vi "RollCalc.vi"(10 "Previous Roll Value":dbl, 11 "Roll Input":dbl) -> (2 "New Roll Value":dbl, 3 "Adjustment to be Made":dbl)   [LabVIEW 2015, in "lv-attitudecontrol.lvlib"]
uses:
  lv-attitudecontrol.lvlib
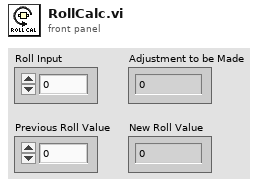
[diagram p1: front panel]
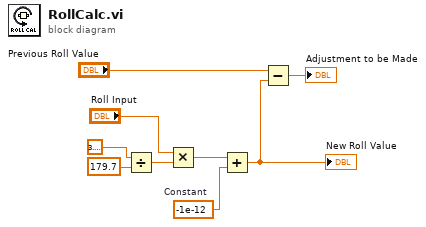
[diagram p0: block diagram]
diagram:
  w7 = -1e-12  # Constant
  n1 = Divide(x=3.141592653589793, y=179.7 ("y 2")) -> (x/y=w5:dbl)
  n2 = Multiply(x="Roll Input", y=w5) -> (x*y=w3:dbl)
  n3 = Add(x=w3, y=w7) -> (x+y=w8:dbl)
  "New Roll Value" <- w8
  n4 = Subtract(x="Previous Roll Value", y=w8) -> (x-y=→"Adjustment to be Made":dbl)
